vi "Laser manager 1.0BETA.vi"() -> ()   [LabVIEW 2014]
uses:
  <vilib>/userdefined/High Color/IMAQdx.ctl
  Typedef/Consumer loop - States.ctl
  Typedef/UI data.ctl
  <vilib>/vision/driver/NI_Vision_Acquisition_Software.lvlib
panel:
  in  "Move":bool
  in  "Absolute Y":dbl caption="Absolute Y [mm]"
  in  "Absolute X":dbl caption="Absolute X [mm]"
  in  "Delta Y":dbl caption="Delta Y [mm]"
  in  "Delta X":dbl caption="Delta X [mm]"
  in  "Move type":enum32{"Step mode", "\"Go to\" mode"}(radio)=enum."\"Go to\" mode"
  in  "Right":bool
  in  "Left":bool
  in  "Up":bool
  in  "Down":bool
  in  "Exit":bool
  out "Image":T1(plugin-control)
  in  "Tab Control":enum32{"Standard operations", "Refill", "Tools"}(tab)
  in  "Main - Open calib":bool
  in  "Go to calib":bool
  in  "Save calib":bool
  in  "Thyratron Bias [kV]":dbl=20.0
  in  "Test Laser":bool
  in  "Frequency [Hz]":u16=1 min=1 max=50 step=1
  in  "Beam Y":dbl=63.0 caption="Y" min=0.1 step=1.0 format="%#_gmm"
  in  "Beam X":dbl=1.0 caption="X" min=0.1 step=1.0 format="%#_gmm"
  in  "How to choose":bool
  in  "Load Pt2":bool
  out "X2":dbl format="%.2fmm"
  out "Y2":dbl format="%.2fmm"
  in  "Load Pt1":bool
  out "X1":dbl format="%.2fmm"
  out "Y1":dbl format="%.2fmm"
  in  "Abort":bool
  in  "Beam Overlap":dbl caption="Lateral Overlap [mm]" min=0.0 max=62.0 step=1.0
  in  "Shots/point":dbl=1.0 min=1.0 max=200.0 step=1.0
  in  "Xspeed":dbl=1.0 caption="X speed [mm/s]" min=0.01 max=100.0 format="%#_3g"
  in  "Irradiate":bool
  out "Pressure":string caption="Pressure [mbar]"
  in  "Refill":bool
  in  "Purge Inert":bool
  in  "Purge Buffer":bool
  in  "Purge Rare":bool
  in  "Purge Halogen":bool
  in  "Set Gas Pressures [mbar]":T2={"Halogen"=80, "Rare"=60, "Buffer "=3160, "Inert"=0}
  in  "Open GPIB interface":bool
  in  "Enable motors":bool
  in  "Find Origin":bool
  in  "Reset ESP":bool
  in  "Tools - Open Calib":bool
  in  "Open Attenuator":bool
  # "Free mode"
  # "LASER MANAGER 1.0 BETA"
  # "written by frax84"
  # "Energy Calibration"
  # "Laser Parameters"
  # "Beam parameters"
  # "Beam size"
  # "Motor path settings"
  # "Irradiation main controls"
  # "Purge Options"
  # "CAUTION\nEach purge operation \nlasts 5 seconds!"
  # "Reading is performed\nevery 5 seconds"
  # "Peripherals comunication"
  # "Motor Utilities"
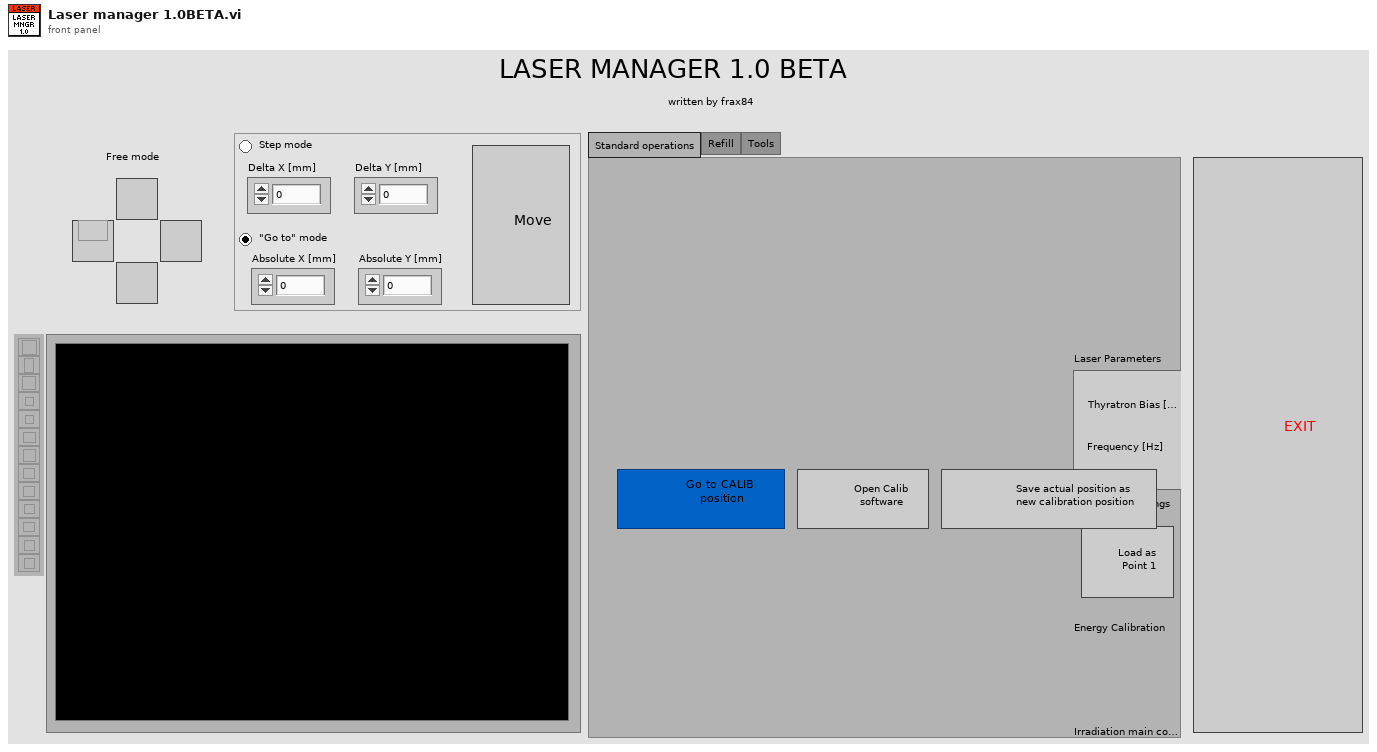
[diagram p1: front panel]
types:
  T1 = typedef "IMAQ Image.ctl" = refnum<image>
  T2 = cluster{"Halogen":u16, "Rare":u16, "Buffer ":u16, "Inert":u16}
  T3 = typedef "UI data.ctl" = cluster{"GPIB Addresses":cluster{"GPIB Motor":i16, "GPIB Laser":string}, "Beam size":cluster{"BeamX":dbl, "BeamY":dbl, "Beam Overlap":dbl}, "Motor speed":cluster{"Xspeed":dbl, " Yspeed":dbl}, "Laser parameters":cluster{"Thyratron Bias":dbl, "Frequency":u16, "Shots/Point":dbl}, "Irradiation points":cluster{"X1":dbl, "Y1":dbl, "X2":dbl, "Y2":dbl}, "Calibration Point":cluster{"Xcalib":dbl, "Ycalib":dbl}}
  T4 = typedef "Consumer loop - States.ctl" = enum16{"Idle", "Read Pressure", "Move up", "Move down", "Move left", "Move right", "Move to", "Move Delta", "Stop Motion", "Go to calib", "Check if move done", "Disable buttons", "Enable buttons", "Irradiation - Stop", "Irradiation - Check points", "Irradiation - Disable buttons", "Irradiation - Init position", "Irradiation - Check if done", "Irradiation - Sweep X", "Irradiation - Check X", "Irradiation - Check Y", "Irradiation - Sweep Y", "Irradiation - Enable buttons"}
  T5 = typedef "Image Type" = u32
  T6 = typedef "IMAQdx.ctl" = refnum<k21>
  T7 = enum8{"Enabled", "Disabled", "Disabled and Grayed Out"}
  T8 = cluster{"Global Rectangle":i32[], "Contours":cluster{"Contour Type":u32, "ROI Type":u32, "Points":i32[]}[]}
  T9 = cluster{"Global Rectangle[0]":i32, "Global Rectangle[1]":i32, "Global Rectangle[2]":i32, "Global Rectangle[3]":i32}
  T10 = cluster{"Consumer loop - States":T4, "Variant":variant}
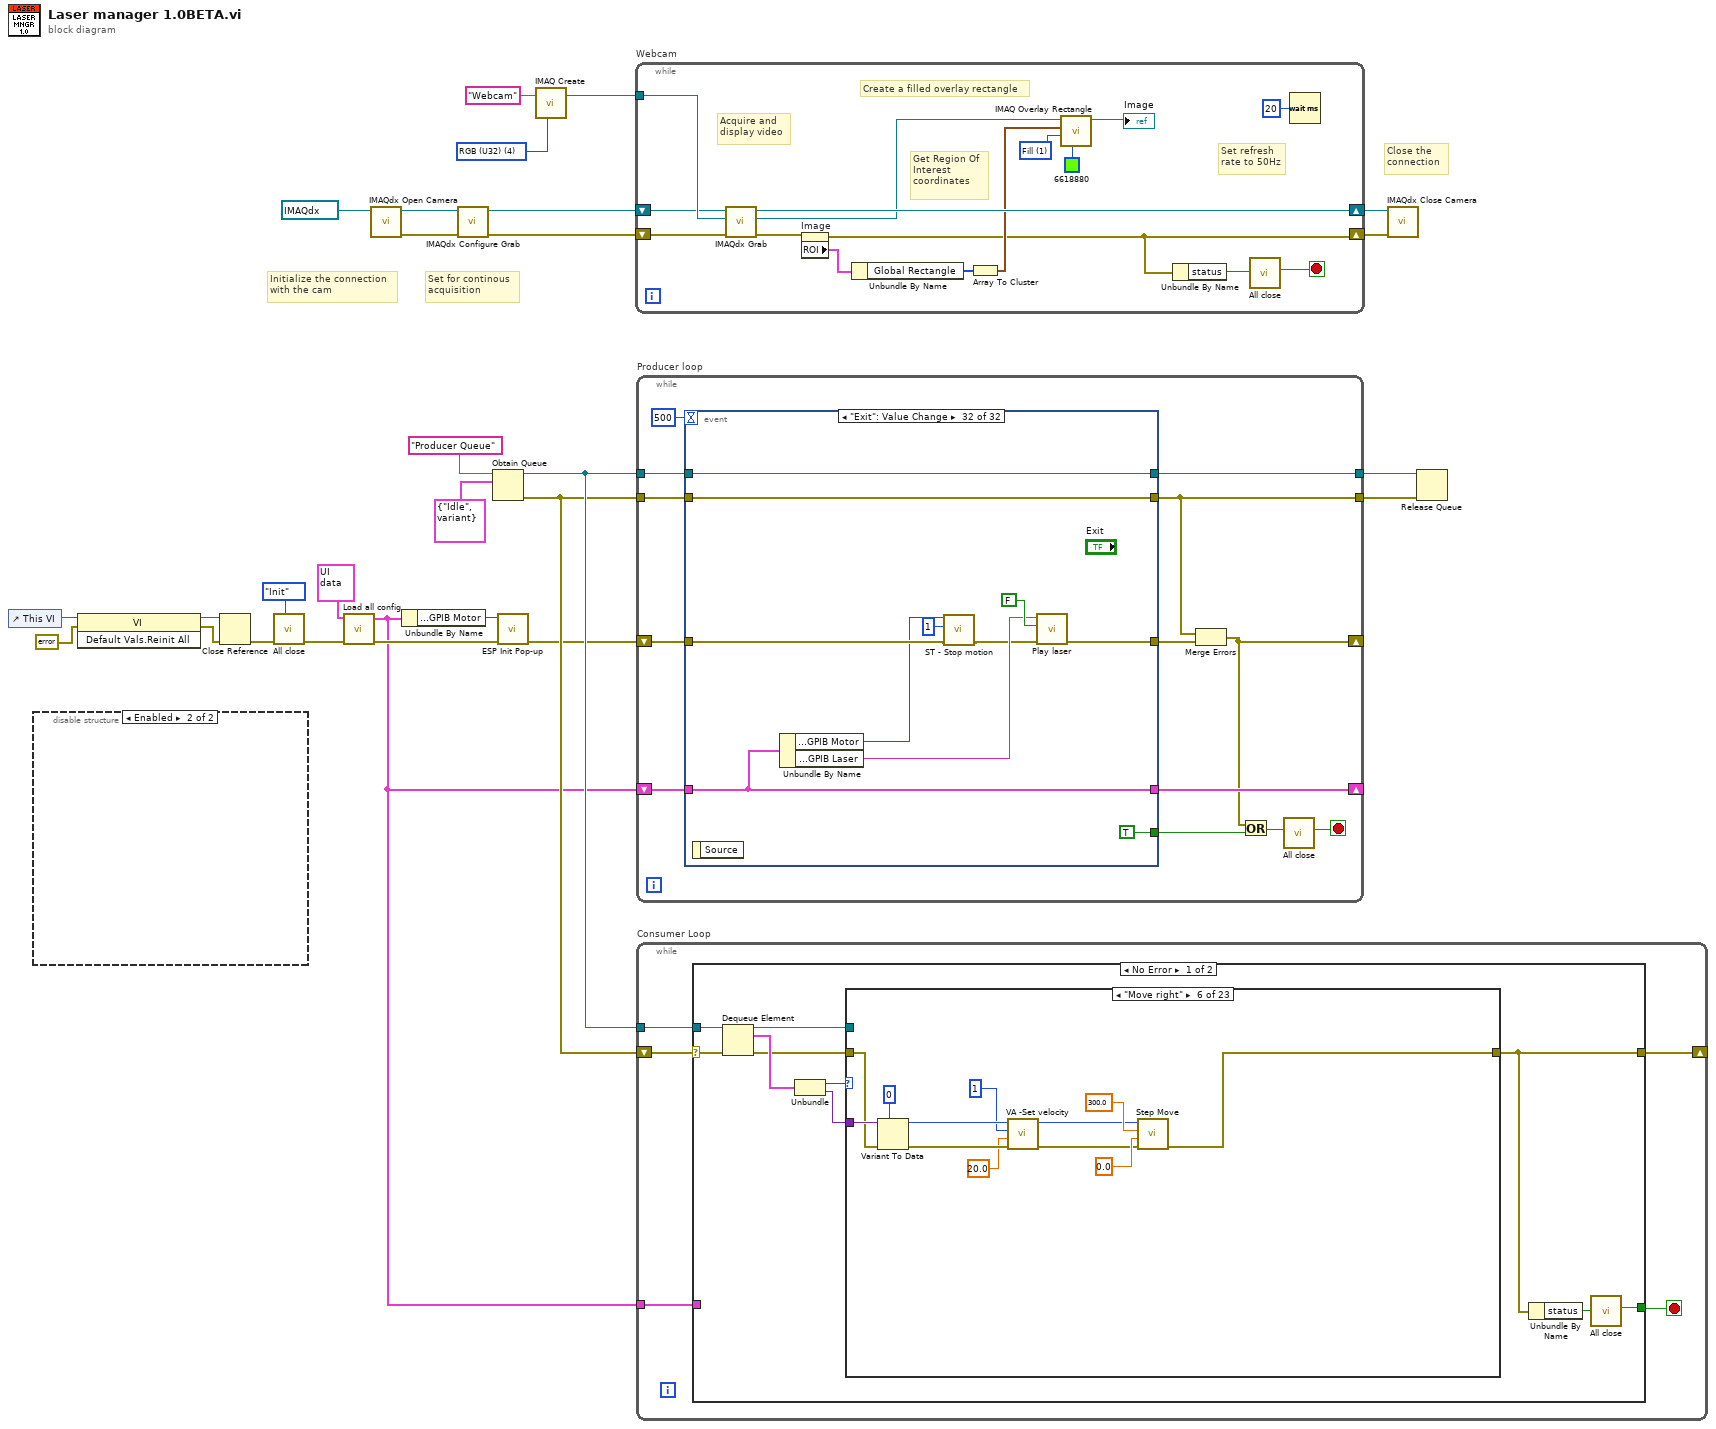
[diagram p0: block diagram]
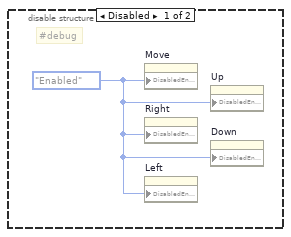
[diagram p2: hidden frame]
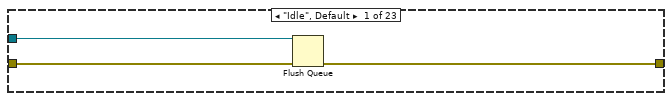
[diagram p3: hidden frame]
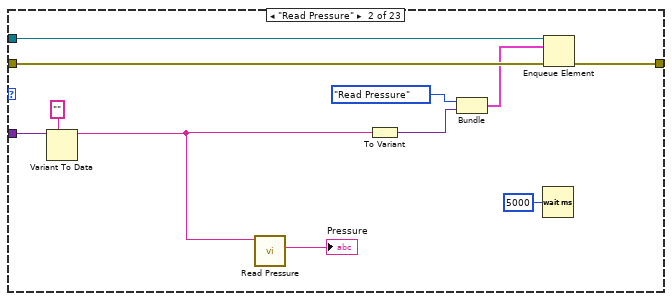
[diagram p4: hidden frame]
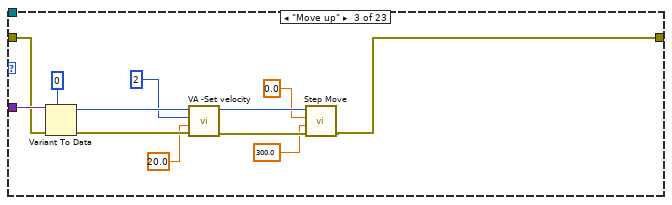
[diagram p5: hidden frame]
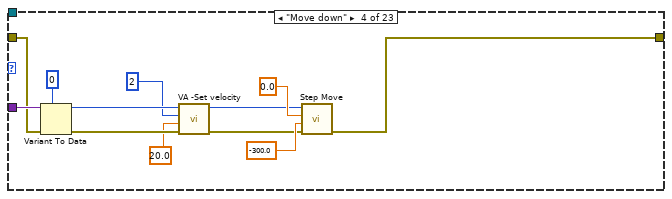
[diagram p6: hidden frame]
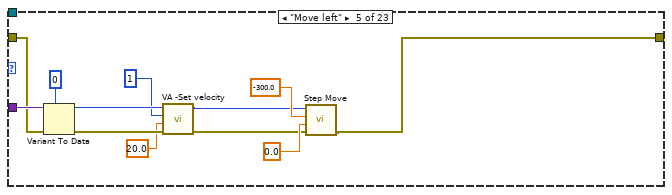
[diagram p7: hidden frame]
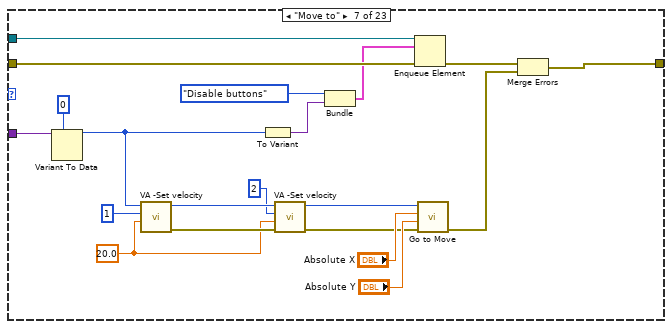
[diagram p8: hidden frame]
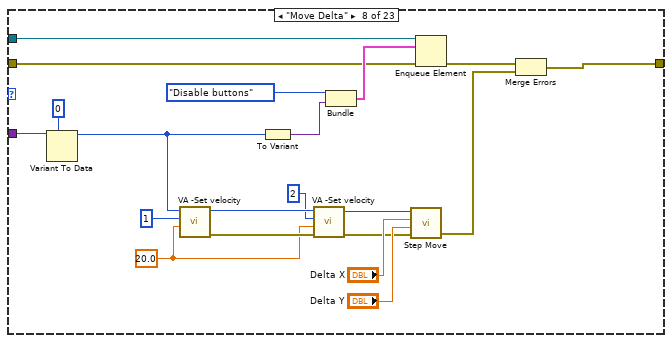
[diagram p9: hidden frame]
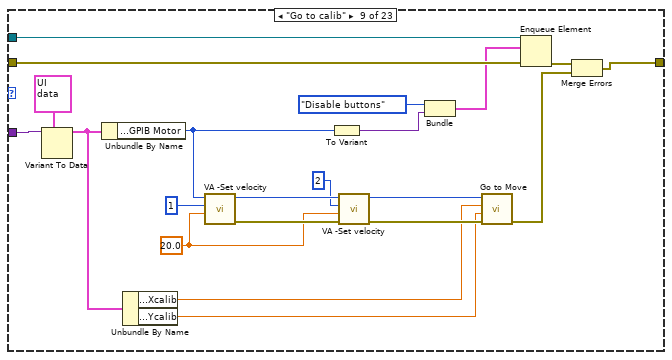
[diagram p10: hidden frame]
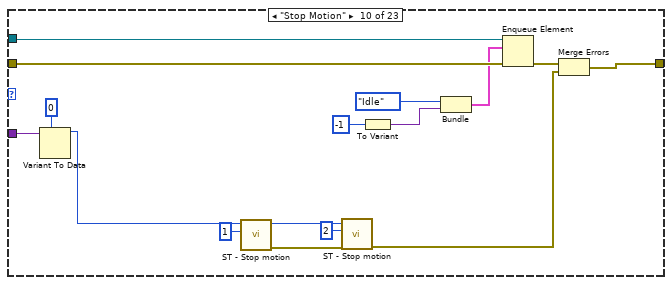
[diagram p11: hidden frame]
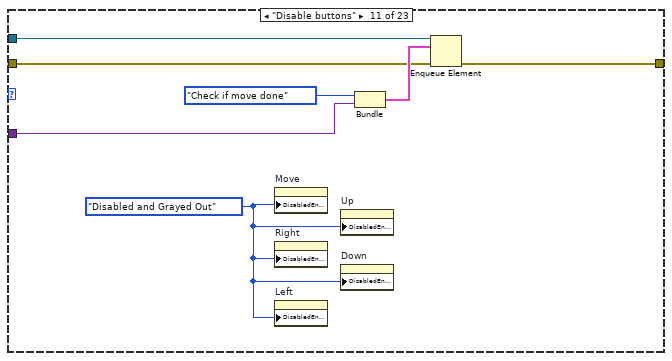
[diagram p12: hidden frame]
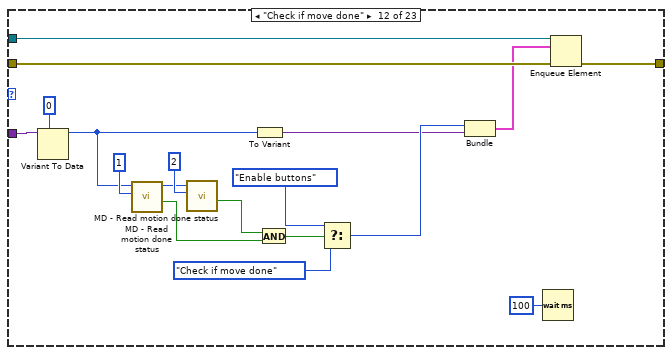
[diagram p13: hidden frame]
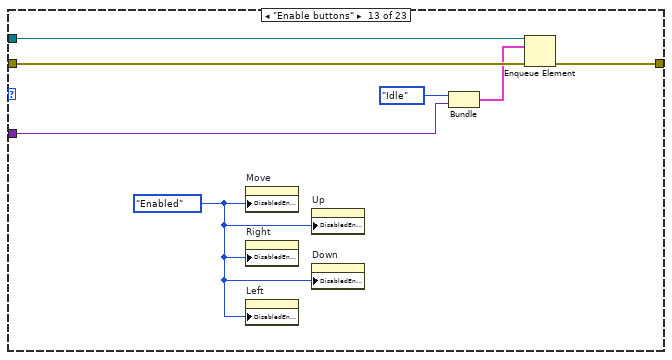
[diagram p14: hidden frame]
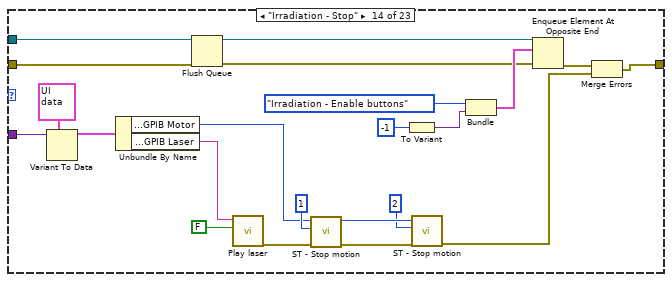
[diagram p15: hidden frame]
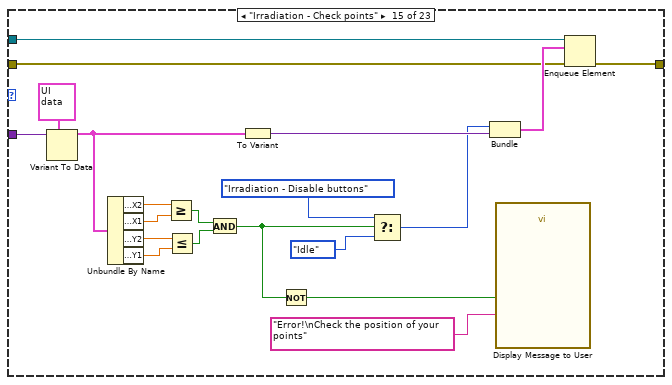
[diagram p16: hidden frame]
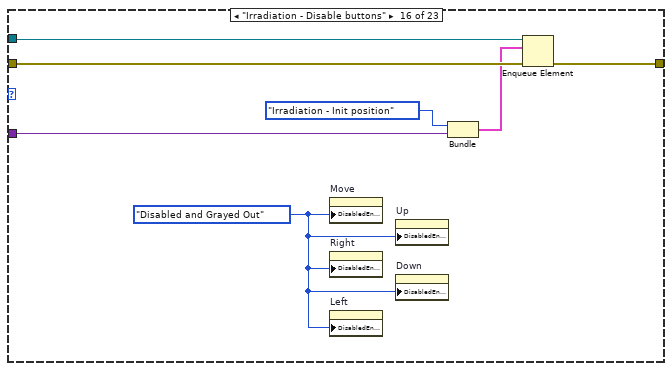
[diagram p17: hidden frame]
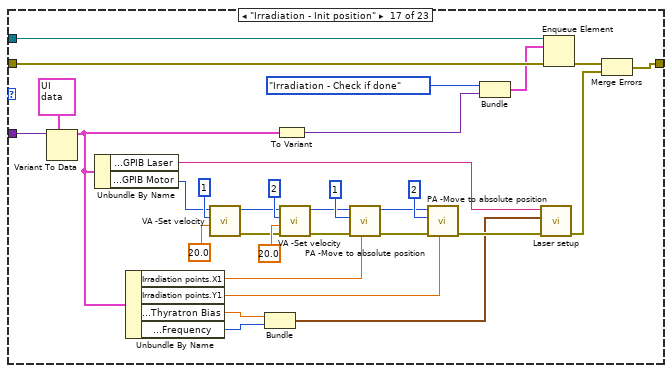
[diagram p18: hidden frame]
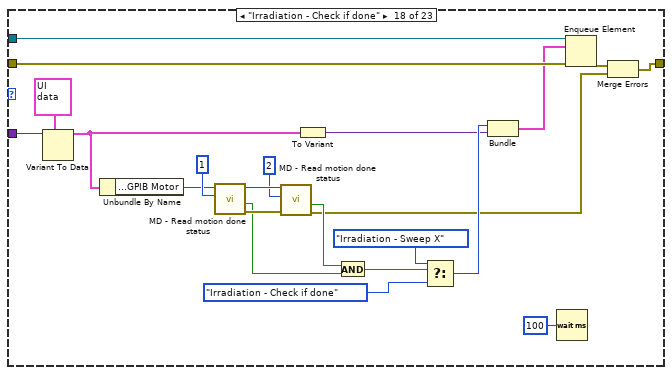
[diagram p19: hidden frame]
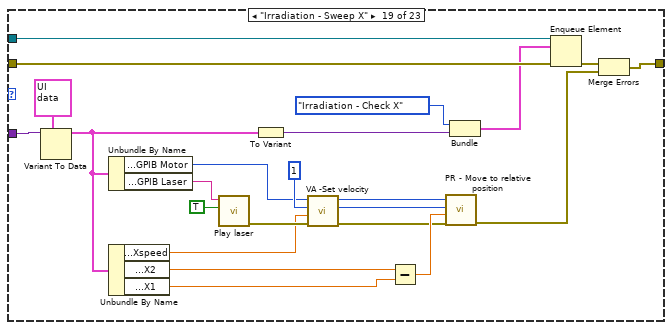
[diagram p20: hidden frame]
diagram:
  w22 = T5 4 items=["Grayscale (U8)", "Grayscale (I16)", "Grayscale (SGL)", "Complex (CSG)", "RGB (U32)", "HSL (U32)", "RGB (U64)", "Grayscale (U16)"] ("Image Type")
  # "Close the \nconnection"
  # "Set for continous\nacquisition"
  # "Initialize the connection\nwith the cam"
  n1 = control-ref of="This VI"() -> (w5:refnum<vi>)
  n2 = disable-structure shown="Enabled" {
    frame Disabled {
      w29 = T7."Enabled" ("Disabled")
      # "#debug"
      n3 = property on="Move" class="Bool"("DisabledEnum"=w29) -> ()  [unwired: 2 in, 2 out]
      n4 = property on="Right" class="Bool (strict)"("DisabledEnum"=w29) -> ()  [unwired: 2 in, 2 out]
      n5 = property on="Left" class="Bool (strict)"("DisabledEnum"=w29) -> ()  [unwired: 2 in, 2 out]
      n6 = property on="Up" class="Bool (strict)"("DisabledEnum"=w29) -> ()  [unwired: 2 in, 2 out]
      n7 = property on="Down" class="Bool (strict)"("DisabledEnum"=w29) -> ()  [unwired: 2 in, 2 out]
    }
    frame Enabled {
    }
  }
  n8 = invoke class="VI" method="Default Vals.Reinit All"(reference=w5, error in=errorcluster {"status"=FALSE, "code"=0, "source"=""} ("Error In")) -> (reference out=w3:refnum<vi>, error out=w4:errorcluster)  [unwired: 1 in, 1 out]
  n9 = Close Reference(reference=w3, error in (no error)=w4) -> (error out=w2:errorcluster)
  n10 = call "All close.vi"("Operation (Check)"=enum16{"Init", "Check"}."Init" ("Operation"), "Error In"=w2) -> ("Error Out"=w8:errorcluster)  [unwired: 8 in, 1 out]
  n11 = call "Load all config.vi"("Error In"=w8, "UI data in"=T3 {"GPIB Addresses"={"GPIB Motor"=2, "GPIB Laser"="3"}, "Beam size"={"BeamX"=1.0, "BeamY"=63.0, "Beam Overlap"=0.0}, "Motor speed"={"Xspeed"=1.0, " Yspeed"=1.0}, "Laser parameters"={"Thyratron Bias"=20.0, "Frequency"=1, "Shots/Point"=1.0}, "Irradiation points"={"X1"=0.0, "Y1"=0.0, "X2"=0.0, "Y2"=0.0}, "Calibration Point"={"Xcalib"=0.0, "Ycalib"=0.0}} ("User Interface data")) -> ("Error Out"=w10:errorcluster, "UI data out"=w9:T3)  [unwired: 8 in]
  n12 = call <vilib>:"IMAQdx Open Camera.vi"("Session In"=T6 "cam1") -> ("error out"=w27:errorcluster, "Session Out"=w28:T6)  [unwired: 9 in]
  n13 = Unbundle By Name(w9) -> ("GPIB Addresses.GPIB Motor"=w13:i16)
  n14 = call <vilib>:"IMAQdx Configure Grab.vi"("error in"=w27, "Session In"=w28) -> ("error out"=w20:errorcluster, "Session Out"=w19:T6)  [unwired: 8 in]
  n15 = Obtain Queue(name (unnamed)="Producer Queue", element data type=cluster{"Consumer loop - States":T4, variant} {"Consumer loop - States"=enum."Idle", variant}) -> (queue out=w17:refnum<queue>, error out=w16:errorcluster)  [unwired: 3 in, 1 out]
  n16 = call "ESP Init Pop-up.vi"("Error In"=w10, "Address / Port in"=w13) -> ("Error Out"=w14:errorcluster)  [unwired: 9 in]
  n17 = call "IMAQ Create"("Image Name"="Webcam", "Image Type"=w22) -> ("New Image"=w23:T1)  [unwired: 3 in, 1 out]
  n18 = while "Webcam" {
    shift-right: [w45] -> w25
    shift-left: w19 -> [w43]
    shift-right: [w31] -> w24
    shift-left: w20 -> [w42]
    tunnel: w23 -> [w44]
    stop <- w32 stop-if-true
    w35 = u32 1 items=["Frame", "Fill", "Highlight"] ("Drawing Mode (Frame)")
    # "Set refresh \nrate to 50Hz"
    # "Get Region Of \nInterest\ncoordinates"
    # "Create a filled overlay rectangle"
    # "Acquire and \ndisplay video"
    n19 = call <vilib>:"IMAQdx Grab.vi"("error in"=w42, "Image In"=w44, "Session In"=w43) -> ("error out"=w41:errorcluster, "Image Out"=w36:T1, "Session Out"=w45:T6)  [unwired: 5 in, 1 out]
    n20 = property on="Image" class="ImageControl"(error in=w41) -> (error out=w31:errorcluster, "ROI"=w40:T8)  [unwired: 1 in, 1 out]
    n21 = Unbundle By Name(w40) -> ("Global Rectangle"=w39:i32[])
    n22 = Array To Cluster(array=w39) -> (cluster=w38:T9)
    n23 = call "IMAQ Overlay Rectangle"("Color"=u32 6618880, "Drawing Mode (Frame)"=w35, "Rectangle"=w38, "Image"=w36) -> ("Image Out"=→"Image":T1)  [unwired: 6 in, 1 out]
    n24 = Unbundle By Name(w31) -> ("status"=w30:bool)
    n25 = call "All close.vi"("Close? (F)"=w30) -> ("Close"=w32:bool)  [unwired: 9 in, 1 out]
    n26 = Wait (ms)(milliseconds to wait=u32 20) -> ()  [unwired: 1 out]
  }
  n27 = while "Producer loop" {
    shift-right: [w49] -> _
    shift-left: w14 -> [w58]
    shift-right: [w56] -> _
    shift-left: w9 -> [w57]
    tunnel: w17 -> [w54]
    tunnel: w16 -> [w53]
    tunnel: [w48] -> w12
    tunnel: [w51] -> w11
    stop <- w46 stop-if-true
    n28 = event shown="[31] \"Exit\": Value Change" {
      selector: _ -> [_ _ _ _ _ _ _ _ _ _ _ _ _ _ _ _ _ _ _ _ _ _ _ _ _ _ _ _ _ _ _ _]
      dyn-events: _ -> [_ _ _ _ _ _ _ _ _ _ _ _ _ _ _ _ _ _ _ _ _ _ _ _ _ _ _ _ _ _ _ _]
      timeout: 500 -> [_ _ _ _ _ _ _ _ _ _ _ _ _ _ _ _ _ _ _ _ _ _ _ _ _ _ _ _ _ _ _ _]
      tunnel: w58 -> [w62 w77 w78 w91 w104 w117 w134 w153 w162 w175 w188 w198 w204 w225 w235 w245 w250 w260 w265 w274 w280 w287 w296 w305 w313 w321 w328 w336 w341 w365 w374 w380]
      tunnel: [w62 w77 w78 w91 w104 w117 w134 w141 w161 w174 w187 w197 w204 w225 w235 w245 w250 w260 w265 w273 w279 w286 w295 w304 w312 w320 w326 w337 w341 w365 w373 w384] -> w50
      tunnel: w57 -> [w61 w68 w83 w97 w108 w123 w131 w147 w159 w172 w182 w192 w200 w224 w231 w241 w253 w259 w268 w271 w277 w284 w294 w303 w311 w318 w327 w335 w345 w362 w372 w385]
      tunnel: [w61 w68 w83 w97 w108 w123 w131 w142 w156 w171 w182 w192 w200 w224 w229 w239 w251 w258 w266 w271 w277 w284 w294 w303 w311 w318 w327 w335 w345 w362 w372 w385] -> w56
      tunnel: [_ _ _ _ _ _ _ _ _ _ _ _ _ _ _ _ _ _ _ _ _ _ _ _ _ _ _ _ _ _ _ TRUE] -> w52
      tunnel: w54 -> [w60 w76 w87 w96 w110 w122 w138 w139 w155 w168 w181 w191 w211 w222 w228 w238 w249 w262 w264 w270 w276 w283 w289 w301 w309 w317 w325 w333 w353 w364 w369 w381]
      tunnel: w53 -> [w59 w75 w86 w95 w109 w121 w135 w140 w154 w167 w180 w190 w212 w223 w227 w237 w248 w261 w263 w269 w275 w282 w288 w300 w308 w316 w324 w332 w352 w363 w367 w382]
      tunnel: [w59 w63 w79 w92 w105 w118 w136 w140 w154 w167 w180 w190 w212 w223 w227 w237 w248 w261 w263 w269 w275 w282 w288 w300 w308 w316 w324 w332 w339 w358 w366 w382] -> w48
      tunnel: [w60 w64 w80 w93 w106 w119 w137 w139 w155 w168 w181 w191 w211 w222 w228 w238 w249 w262 w264 w270 w276 w283 w289 w301 w309 w317 w325 w333 w340 w359 w368 w381] -> w51
      event Timeout {
        # "Needed if error occurs"
        n29 = event-data() -> ()  [unwired: 1 in, 1 out]
      }
      event "Move": Value Change {
        n30 = event-data() -> ()  [unwired: 1 in, 1 out]
        n31 = Unbundle By Name(w68) -> ("GPIB Addresses.GPIB Motor"=w67:i16)
        n32 = Equal?(x="Move type", y=enum32{"Step mode", "\"Go to\" mode"}."\"Go to\" mode") -> (x = y?=w72:bool)
        n33 = To Variant(anything=w67) -> (Variant=w66:variant)
        n34 = Select(t=Consumer_loop_-_States."Move to" ("Consumer loop - States"), s=w72, f=Consumer_loop_-_States."Move Delta") -> (s? t:f=w71:T4)
        n35 = Bundle("f"=w71, "Variant"=w66) -> (w65:cluster{"f":T4, "Variant":variant})  [unwired: 1 in]
        n36 = Enqueue Element(queue=w76, element=w65, error in (no error)=w75) -> (queue out=w64:refnum<queue>, error out=w63:errorcluster)  [unwired: 1 in, 1 out]
      }
      event "Up": Value Change {
        n37 = event-data() -> ("NewVal"=w90:bool)  [unwired: 1 in]
        n38 = Unbundle By Name(w83) -> ("GPIB Addresses.GPIB Motor"=w81:i16)
        n39 = To Variant(anything=w81) -> (Variant=w82:variant)
        n40 = Select(t=Consumer_loop_-_States."Move up", s=w90, f=Consumer_loop_-_States."Stop Motion" ("Consumer loop - States")) -> (s? t:f=w85:T4)
        n41 = Bundle("Consumer loop - States"=w85, "Variant"=w82) -> (w84:T10)  [unwired: 1 in]
        n42 = Enqueue Element(queue=w87, element=w84, error in (no error)=w86) -> (queue out=w80:refnum<queue>, error out=w79:errorcluster)  [unwired: 1 in, 1 out]
      }
      event "Down": Value Change {
        n43 = event-data() -> ("NewVal"=w94:bool)  [unwired: 1 in]
        n44 = Unbundle By Name(w97) -> ("GPIB Addresses.GPIB Motor"=w98:i16)
        n45 = To Variant(anything=w98) -> (Variant=w99:variant)
        n46 = Select(t=Consumer_loop_-_States."Move down", s=w94, f=Consumer_loop_-_States."Stop Motion" ("Consumer loop - States")) -> (s? t:f=w101:T4)
        n47 = Bundle("Consumer loop - States"=w101, "Variant"=w99) -> (w100:T10)  [unwired: 1 in]
        n48 = Enqueue Element(queue=w96, element=w100, error in (no error)=w95) -> (queue out=w93:refnum<queue>, error out=w92:errorcluster)  [unwired: 1 in, 1 out]
      }
      event "Left": Value Change {
        n49 = event-data() -> ("NewVal"=w107:bool)  [unwired: 1 in]
        n50 = Unbundle By Name(w108) -> ("GPIB Addresses.GPIB Motor"=w116:i16)
        n51 = To Variant(anything=w116) -> (Variant=w115:variant)
        n52 = Select(t=Consumer_loop_-_States."Move left", s=w107, f=Consumer_loop_-_States."Stop Motion" ("Consumer loop - States")) -> (s? t:f=w113:T4)
        n53 = Bundle("Consumer loop - States"=w113, "Variant"=w115) -> (w114:T10)  [unwired: 1 in]
        n54 = Enqueue Element(queue=w110, element=w114, error in (no error)=w109) -> (queue out=w106:refnum<queue>, error out=w105:errorcluster)  [unwired: 1 in, 1 out]
      }
      event "Right": Value Change {
        n55 = event-data() -> ("NewVal"=w120:bool)  [unwired: 1 in]
        n56 = Unbundle By Name(w123) -> ("GPIB Addresses.GPIB Motor"=w129:i16)
        n57 = To Variant(anything=w129) -> (Variant=w128:variant)
        n58 = Select(t=Consumer_loop_-_States."Move right", s=w120, f=Consumer_loop_-_States."Stop Motion" ("Consumer loop - States")) -> (s? t:f=w126:T4)
        n59 = Bundle("Consumer loop - States"=w126, "Variant"=w128) -> (w127:T10)  [unwired: 1 in]
        n60 = Enqueue Element(queue=w122, element=w127, error in (no error)=w121) -> (queue out=w119:refnum<queue>, error out=w118:errorcluster)  [unwired: 1 in, 1 out]
      }
      event "Go to calib": Value Change {
        n61 = event-data() -> ()  [unwired: 1 in, 1 out]
        n62 = To Variant(anything=w131) -> (Variant=w130:variant)
        n63 = Bundle("Consumer loop - States"=Consumer_loop_-_States."Go to calib", "Variant"=w130) -> (w133:T10)  [unwired: 1 in]
        n64 = Enqueue Element(queue=w138, element=w133, error in (no error)=w135) -> (queue out=w137:refnum<queue>, error out=w136:errorcluster)  [unwired: 1 in, 1 out]
      }
      event "Save calib": Value Change {
        n65 = event-data() -> ()  [unwired: 1 in, 1 out]
        n66 = Unbundle By Name(w147) -> ("GPIB Addresses.GPIB Motor"=w152:i16)
        n67 = call "TP - Read actual position.vi"("error in"=w153, "Axis"=i8 1, "Address / Port"=w152) -> ("error out"=w150:errorcluster, "Query the current actual\nposition - read"=w146:dbl, "Address / Port dup"=w149:i16)  [unwired: 5 in, 1 out]
        n68 = call "TP - Read actual position.vi"("error in"=w150, "Axis"=i8 2, "Address / Port"=w149) -> ("error out"=w144:errorcluster, "Query the current actual\nposition - read"=w145:dbl)  [unwired: 5 in, 2 out]
        n69 = Bundle By Name(cluster=w147, "Calibration Point.Ycalib"=w145, "Calibration Point.Xcalib"=w146) -> (w143:T3)
        n70 = call "Save calib config.vi"("Error In"=w144, "UI data in"=w143) -> ("Error Out"=w141:errorcluster, "UI data out"=w142:T3)  [unwired: 8 in]
      }
      event "Load Pt1": Value Change {
        n71 = event-data() -> ()  [unwired: 1 in, 1 out]
        n72 = Unbundle By Name(w159) -> ("GPIB Addresses.GPIB Motor"=w160:i16)
        n73 = call "TP - Read actual position.vi"("error in"=w162, "Axis"=i8 1, "Address / Port"=w160) -> ("error out"=w165:errorcluster, "Query the current actual\nposition - read"=w158:dbl, "Address / Port dup"=w166:i16)  [unwired: 5 in, 1 out]
        "X1" <- w158
        n74 = call "TP - Read actual position.vi"("error in"=w165, "Axis"=i8 2, "Address / Port"=w166) -> ("error out"=w161:errorcluster, "Query the current actual\nposition - read"=w157:dbl)  [unwired: 5 in, 2 out]
        "Y1" <- w157
        n75 = Bundle By Name(cluster=w159, "Irradiation points.Y1"=w157, "Irradiation points.X1"=w158) -> (w156:T3)
      }
      event "Load Pt2": Value Change {
        n76 = event-data() -> ()  [unwired: 1 in, 1 out]
        n77 = Unbundle By Name(w172) -> ("GPIB Addresses.GPIB Motor"=w173:i16)
        n78 = call "TP - Read actual position.vi"("error in"=w175, "Axis"=i8 1, "Address / Port"=w173) -> ("error out"=w178:errorcluster, "Query the current actual\nposition - read"=w170:dbl, "Address / Port dup"=w179:i16)  [unwired: 5 in, 1 out]
        "X2" <- w170
        n79 = call "TP - Read actual position.vi"("error in"=w178, "Axis"=i8 2, "Address / Port"=w179) -> ("error out"=w174:errorcluster, "Query the current actual\nposition - read"=w169:dbl)  [unwired: 5 in, 2 out]
        "Y2" <- w169
        n80 = Bundle By Name(cluster=w172, "Irradiation points.Y2"=w169, "Irradiation points.X2"=w170) -> (w171:T3)
      }
      event "Tools - Open Calib", "Main - Open calib": Value Change {
        n81 = event-data() -> ()  [unwired: 1 in, 1 out]
        n82 = call <vilib>:"Application Directory.vi"() -> ("Application Directory"=w186:path)
        n83 = Build Path(base path=w186, name or relative path="External software\\Thorlabs\\Optical Power Meter Utility.exe" ("command line")) -> (appended path=w185:path)
        n84 = Path To String(path=w185) -> (string=w183:string)
        n85 = call <vilib>:"System Exec.vi"("wait until completion? (T)"=FALSE, "error in (no error)"=w188, "command line"=w183) -> ("error out"=w187:errorcluster)  [unwired: 5 in, 3 out]
      }
      event "Open Attenuator": Value Change {
        n86 = event-data() -> ()  [unwired: 1 in, 1 out]
        n87 = call <vilib>:"Application Directory.vi"() -> ("Application Directory"=w196:path)
        n88 = Build Path(base path=w196, name or relative path="External software\\Coherent\\CohrAttenuatorApp.exe" ("command line")) -> (appended path=w195:path)
        n89 = Path To String(path=w195) -> (string=w193:string)
        n90 = call <vilib>:"System Exec.vi"("wait until completion? (T)"=FALSE, "error in (no error)"=w198, "command line"=w193) -> ("error out"=w197:errorcluster)  [unwired: 5 in, 3 out]
      }
      event "Open GPIB interface": Value Change {
        n91 = event-data() -> ()  [unwired: 1 in, 1 out]
        n92 = call <vilib>:"Application Directory.vi"() -> ("Application Directory"=w203:path)
        n93 = Build Path(base path=w203, name or relative path="Utilities\\GPIB \nSimple Interface.vi") -> (appended path=w201:path)
        n94 = Open VI Reference(vi path=w201) -> (vi reference=w209:refnum<vi>, error out=w206:errorcluster)  [unwired: 5 in]
        n95 = property class="VI"(reference=w209, error in=w206, "Front Panel Window:Open"=TRUE) -> (reference out=w208:refnum<vi>, error out=w205:errorcluster)
        n96 = invoke class="VI" method="Run VI"(reference=w208, error in=w205, "Wait until done"=FALSE) -> ()  [unwired: 2 in, 5 out]
      }
      event "How to choose": Value Change {
        n97 = event-data() -> ()  [unwired: 1 in, 1 out]
        n98 = call <vilib>:"Application Directory.vi"() -> ("Application Directory"=w215:path)
        n99 = Build Path(base path=w215, name or relative path="SubVIs\\How to.vi") -> (appended path=w213:path)
        n100 = Open VI Reference(vi path=w213) -> (vi reference=w220:refnum<vi>, error out=w217:errorcluster)  [unwired: 5 in]
        n101 = property class="VI"(reference=w220, error in=w217, "Front Panel Window:Open"=TRUE) -> (reference out=w219:refnum<vi>, error out=w216:errorcluster)
        n102 = invoke class="VI" method="Run VI"(reference=w219, error in=w216, "Wait until done"=FALSE) -> ()  [unwired: 2 in, 5 out]
      }
      event "Shots/point": Value Change {
        n103 = event-data() -> ()  [unwired: 1 in, 1 out]
        n104 = Unbundle By Name(w231) -> ("Beam size.BeamX"=w234:dbl, "Laser parameters.Frequency"=w233:u16)
        n105 = Multiply(x=w234, y=w233) -> (x*y=w232:dbl)
        n106 = Divide(x=w232, y="Shots/point") -> (x/y=w226:dbl)
        n107 = Bundle By Name(cluster=w231, "Motor speed.Xspeed"=w226, "Laser parameters.Shots/Point"="Shots/point") -> (w229:T3)
        n108 = local write "Xspeed"(w226) -> ()
      }
      event "Xspeed": Value Change {
        n109 = event-data() -> ()  [unwired: 1 in, 1 out]
        n110 = Unbundle By Name(w241) -> ("Beam size.BeamX"=w244:dbl, "Laser parameters.Frequency"=w243:u16)
        n111 = Multiply(x=w244, y=w243) -> (x*y=w242:dbl)
        n112 = Divide(x=w242, y="Xspeed") -> (x/y=w236:dbl)
        n113 = local write "Shots/point"(w236) -> ()
        n114 = Bundle By Name(cluster=w241, "Laser parameters.Shots/Point"=w236, "Motor speed.Xspeed"="Xspeed") -> (w239:T3)
      }
      event "Frequency [Hz]", "Beam X": Value Change {
        n115 = event-data() -> ()  [unwired: 1 in, 1 out]
        n116 = Unbundle By Name(w253) -> ("Laser parameters.Shots/Point"=w254:dbl)
        n117 = Multiply(x="Frequency [Hz]", y="Beam X") -> (x*y=w255:dbl)
        n118 = Divide(x=w255, y=w254) -> (x/y=w247:dbl)
        n119 = local write "Xspeed"(w247) -> ()
        n120 = Bundle By Name(cluster=w253, "Laser parameters.Frequency"="Frequency [Hz]", "Beam size.BeamX"="Beam X", "Motor speed.Xspeed"=w247) -> (w251:T3)
      }
      event "Beam Overlap", "Beam Y": Value Change {
        n121 = event-data() -> ()  [unwired: 1 in, 1 out]
        n122 = Bundle By Name(cluster=w259, "Beam size.BeamY"="Beam Y", "Beam size.Beam Overlap"="Beam Overlap") -> (w258:T3)
      }
      event "Thyratron Bias [kV]": Value Change {
        n123 = event-data() -> ()  [unwired: 1 in, 1 out]
        n124 = Bundle By Name(cluster=w268, "Laser parameters.Thyratron Bias"="Thyratron Bias [kV]") -> (w266:T3)
      }
      event "Find Origin": Value Change {
        n125 = event-data() -> ()  [unwired: 1 in, 1 out]
        n126 = Unbundle By Name(w271) -> ("GPIB Addresses.GPIB Motor"=w272:i16)
        n127 = call "Find Origin.vi"("Error In"=w274, "Address / Port"=w272) -> ("Error Out"=w273:errorcluster)  [unwired: 8 in, 1 out]
      }
      event "Enable motors": Value Change {
        n128 = event-data() -> ()  [unwired: 1 in, 1 out]
        n129 = Unbundle By Name(w277) -> ("GPIB Addresses.GPIB Motor"=w278:i16)
        n130 = call "Enable Motor.vi"("Error In"=w280, "On/Off"=enum16{"On", "Off"}."On", "Address / Port"=w278) -> ("Error Out"=w279:errorcluster)  [unwired: 7 in, 1 out]
      }
      event "Reset ESP": Value Change {
        n131 = event-data() -> ()  [unwired: 1 in, 1 out]
        n132 = Unbundle By Name(w284) -> ("GPIB Addresses.GPIB Motor"=w285:i16)
        n133 = call "RS - Reset the controller.vi"("error in"=w287, "Address / Port"=w285) -> ("error out"=w286:errorcluster)  [unwired: 6 in, 1 out]
      }
      event "Test Laser": Value Change {
        n134 = event-data() -> ("NewVal"=w297:bool)  [unwired: 1 in]
        n135 = Unbundle By Name(w294) -> ("GPIB Addresses.GPIB Laser"=w293:string, "Laser parameters.Thyratron Bias"=w292:dbl, "Laser parameters.Frequency"=w291:u16)
        n136 = Bundle("Thyratron Bias"=w292, "Frequency"=w291) -> (w290:cluster{"Thyratron Bias":dbl, "Frequency":u16})  [unwired: 1 in]
        n137 = call "Laser setup.vi"("Error In"=w296, "Laser Parameters"=w290, "GPIB Address"=w293) -> ("Error Out"=w298:errorcluster, "GPIB Address out"=w299:string)  [unwired: 7 in]
        n138 = call "Play laser.vi"("Error In"=w298, "Laser On"=w297, "GPIB Address"=w299) -> ("Error Out"=w295:errorcluster)  [unwired: 7 in, 1 out]
      }
      event "Purge Halogen": Value Change {
        n139 = event-data() -> ()  [unwired: 1 in, 1 out]
        n140 = Unbundle By Name(w303) -> ("GPIB Addresses.GPIB Laser"=w302:string)
        n141 = call "Purge Line.vi"("Error In"=w305, "Gas"=enum16{"Halogen", "Rare", "Buffer", "Inert"}."Halogen", "GPIB Address"=w302) -> ("Error Out"=w304:errorcluster)  [unwired: 7 in, 1 out]
        n142 = Wait (ms)(milliseconds to wait=u32 6000) -> ()  [unwired: 1 out]
      }
      event "Purge Rare": Value Change {
        n143 = event-data() -> ()  [unwired: 1 in, 1 out]
        n144 = Unbundle By Name(w311) -> ("GPIB Addresses.GPIB Laser"=w310:string)
        n145 = call "Purge Line.vi"("Error In"=w313, "Gas"=enum16{"Halogen", "Rare", "Buffer", "Inert"}."Rare", "GPIB Address"=w310) -> ("Error Out"=w312:errorcluster)  [unwired: 7 in, 1 out]
        n146 = Wait (ms)(milliseconds to wait=u32 6000) -> ()  [unwired: 1 out]
      }
      event "Purge Buffer": Value Change {
        n147 = event-data() -> ()  [unwired: 1 in, 1 out]
        n148 = Unbundle By Name(w318) -> ("GPIB Addresses.GPIB Laser"=w319:string)
        n149 = call "Purge Line.vi"("Error In"=w321, "Gas"=enum16{"Halogen", "Rare", "Buffer", "Inert"}."Buffer", "GPIB Address"=w319) -> ("Error Out"=w320:errorcluster)  [unwired: 7 in, 1 out]
        n150 = Wait (ms)(milliseconds to wait=u32 6000) -> ()  [unwired: 1 out]
      }
      event "Purge Inert": Value Change {
        n151 = event-data() -> ()  [unwired: 1 in, 1 out]
        n152 = Unbundle By Name(w327) -> ("GPIB Addresses.GPIB Laser"=w329:string)
        n153 = call "Purge Line.vi"("Error In"=w328, "Gas"=enum16{"Halogen", "Rare", "Buffer", "Inert"}."Inert", "GPIB Address"=w329) -> ("Error Out"=w326:errorcluster)  [unwired: 7 in, 1 out]
        n154 = Wait (ms)(milliseconds to wait=u32 6000) -> ()  [unwired: 1 out]
      }
      event "Refill": Value Change {
        n155 = event-data() -> ()  [unwired: 1 in, 1 out]
        n156 = Unbundle By Name(w335) -> ("GPIB Addresses.GPIB Laser"=w334:string)
        n157 = call "New Fill.vi"("Error In"=w336, "Gas settings"="Set Gas Pressures [mbar]", "GPIB Address"=w334) -> ("Error Out"=w337:errorcluster)  [unwired: 7 in, 1 out]
      }
      event "Tab Control": Value Change {
        # "If the Refill tab is chosen pressure is read every 5 seconds"
        n158 = event-data() -> ()  [unwired: 1 in, 1 out]
        n159 = Unbundle By Name(w345) -> ("GPIB Addresses.GPIB Laser"=w344:string)
        n160 = Equal?(x="Tab Control", y=enum32{"Standard operations", "Refill", "Tools"}."Refill") -> (x = y?=w349:bool)
        n161 = To Variant(anything=w344) -> (Variant=w343:variant)
        n162 = Select(t=Consumer_loop_-_States."Read Pressure" ("Consumer loop - States"), s=w349, f=Consumer_loop_-_States."Idle") -> (s? t:f=w346:T4)
        n163 = Bundle("f"=w346, "Variant"=w343) -> (w342:cluster{"f":T4, "Variant":variant})  [unwired: 1 in]
        n164 = Enqueue Element(queue=w353, element=w342, error in (no error)=w352) -> (queue out=w340:refnum<queue>, error out=w339:errorcluster)  [unwired: 1 in, 1 out]
      }
      event "Irradiate": Value Change {
        n165 = event-data() -> ("NewVal"=w357:bool)  [unwired: 1 in]
        n166 = To Variant(anything=w362) -> (Variant=w361:variant)
        n167 = Select(t=Consumer_loop_-_States."Irradiation - Check points" ("Consumer loop - States"), s=w357, f=Consumer_loop_-_States."Irradiation - Stop") -> (s? t:f=w355:T4)
        n168 = Bundle("f"=w355, "Variant"=w361) -> (w360:cluster{"f":T4, "Variant":variant})  [unwired: 1 in]
        n169 = Enqueue Element(queue=w364, element=w360, error in (no error)=w363) -> (queue out=w359:refnum<queue>, error out=w358:errorcluster)  [unwired: 1 in, 1 out]
      }
      event "Abort": Value Change {
        n170 = event-data() -> ()  [unwired: 1 in, 1 out]
        n171 = Unbundle By Name(w372) -> ("GPIB Addresses.GPIB Motor"=w371:i16, "GPIB Addresses.GPIB Laser"=w370:string)
        n172 = Flush Queue(queue=w369, error in (no error)=w367) -> (queue out=w368:refnum<queue>, error out=w366:errorcluster)  [unwired: 1 out]
        n173 = call "AB - Abort Motion.vi"("error in"=w374, "Address / Port"=w371) -> ("error out"=w376:errorcluster)  [unwired: 9 in]
        n174 = call "Play laser.vi"("Error In"=w376, "Laser On"=FALSE, "GPIB Address"=w370) -> ("Error Out"=w373:errorcluster)  [unwired: 7 in, 1 out]
      }
      event "Exit": Value Change {
        n175 = event-data() -> ()  [unwired: 1 in, 1 out]
        n176 = Unbundle By Name(w385) -> ("GPIB Addresses.GPIB Motor"=w378:i16, "GPIB Addresses.GPIB Laser"=w383:string)
        n177 = call "ST - Stop motion.vi"("error in"=w380, "Axis"=i8 1, "Address / Port"=w378) -> ("error out"=w379:errorcluster)  [unwired: 6 in, 2 out]
        n178 = call "Play laser.vi"("Error In"=w379, "Laser On"=FALSE, "GPIB Address"=w383) -> ("Error Out"=w384:errorcluster)  [unwired: 7 in, 1 out]
      }
    }
    n179 = Merge Errors(w48, w50) -> (w49:errorcluster)
    n180 = Or(x=w49, y=w52) -> (x .or. y?=w47:bool)
    n181 = call "All close.vi"("Close? (F)"=w47) -> ("Close"=w46:bool)  [unwired: 9 in, 1 out]
  }
  n182 = while "Consumer Loop" {
    tunnel: w17 -> [w392]
    shift-right: [w391] -> _
    shift-left: w16 -> [w390]
    tunnel: w9 -> [w388]
    stop <- w389 stop-if-true
    n183 = case shown="No Error" w390 {
      selector: w390 -> [w396 w778]
      tunnel: w392 -> [w402 _]
      tunnel: [w394 w775] -> w391
      tunnel: [w395 TRUE] -> w389
      tunnel: w388 -> [_ w781]
      frame No Error {
        n184 = Dequeue Element(queue=w402, error in (no error)=w396) -> (queue out=w398:refnum<queue>, element=w401:cluster{"Consumer loop - States":T4, variant}, error out=w399:errorcluster)  [unwired: 1 in, 1 out]
        n185 = Unbundle(w401) -> ("Consumer loop - States"=w400:T4, w397:variant)
        n186 = case shown="\"Move right\"" w400 {
          tunnel: w399 -> [w404 w414 w426 w438 w450 w462 w479 w497 w512 w541 w544 w558 w572 w575 w611 w620 w630 w672 w688 w707 w733 w762 w770]
          tunnel: w398 -> [w405 w415 _ _ _ _ w480 w498 w513 w540 w545 w559 w573 w585 w612 w621 w631 w673 w689 w706 w732 w763 w769]
          tunnel: w397 -> [_ w410 w428 w439 w451 w463 w482 w502 w525 w539 w543 w565 w568 w589 w615 w616 w640 w675 w691 w714 w738 w764 w767]
          tunnel: [w403 w406 w419 w429 w442 w455 w474 w494 w506 w531 w542 w549 w567 w588 w602 w619 w623 w657 w681 w700 w726 w760 w768] -> w394
          frame "Idle", Default {
            n187 = Flush Queue(queue=w405, error in (no error)=w404) -> (error out=w403:errorcluster)  [unwired: 2 out]
          }
          frame "Read Pressure" {
            n188 = Variant To Data(type="" ("Instrument GPIB Addresses.GPIB Laser"), Variant=w410) -> (data=w407:string)  [unwired: 1 in, 1 out]
            n189 = call "Read Pressure.vi"("GPIB Address"=w407) -> ("Pressure [mbar]"=→"Pressure":string)  [unwired: 8 in, 2 out]
            n190 = To Variant(anything=w407) -> (Variant=w412:variant)
            n191 = Bundle("Consumer loop - States"=Consumer_loop_-_States."Read Pressure", "Variant"=w412) -> (w411:T10)  [unwired: 1 in]
            n192 = Wait (ms)(milliseconds to wait=u32 5000) -> ()  [unwired: 1 out]
            n193 = Enqueue Element(queue=w415, element=w411, error in (no error)=w414) -> (error out=w406:errorcluster)  [unwired: 1 in, 2 out]
          }
          frame "Move up" {
            n194 = Variant To Data(error in=w426, type=i16 0 ("Address / Port"), Variant=w428) -> (data=w424:i16, error out=w425:errorcluster)
            n195 = call "VA -Set velocity.vi"("error in"=w425, "Velocity\nset"=20.0 ("Velocity\nset"), "Axis #"=i8 2, "Address / Port"=w424) -> ("error out"=w421:errorcluster, "Address / Port dup"=w420:i16)  [unwired: 4 in, 2 out]
            n196 = call "Step Move.vi"("Error In"=w421, "Delta Y"=300.0 ("Move to travel limit\nset (+ or - )"), "Delta X"=0.0, "Address/Port in"=w420) -> ("Error Out"=w419:errorcluster)  [unwired: 6 in, 1 out]
          }
          frame "Move down" {
            n197 = Variant To Data(error in=w438, type=i16 0 ("Address / Port"), Variant=w439) -> (data=w437:i16, error out=w436:errorcluster)
            n198 = call "VA -Set velocity.vi"("error in"=w436, "Velocity\nset"=20.0 ("Velocity\nset"), "Axis #"=i8 2, "Address / Port"=w437) -> ("error out"=w430:errorcluster, "Address / Port dup"=w431:i16)  [unwired: 4 in, 2 out]
            n199 = call "Step Move.vi"("Error In"=w430, "Delta Y"=-300.0 ("Move to travel limit\nset (+ or - )"), "Delta X"=0.0, "Address/Port in"=w431) -> ("Error Out"=w429:errorcluster)  [unwired: 6 in, 1 out]
          }
          frame "Move left" {
            n200 = Variant To Data(error in=w450, type=i16 0 ("Address / Port"), Variant=w451) -> (data=w448:i16, error out=w449:errorcluster)
            n201 = call "VA -Set velocity.vi"("error in"=w449, "Velocity\nset"=20.0 ("Velocity\nset"), "Axis #"=i8 1, "Address / Port"=w448) -> ("error out"=w441:errorcluster, "Address / Port dup"=w443:i16)  [unwired: 4 in, 2 out]
            n202 = call "Step Move.vi"("Error In"=w441, "Delta Y"=0.0 ("Move to travel limit\nset (+ or - )"), "Delta X"=-300.0, "Address/Port in"=w443) -> ("Error Out"=w442:errorcluster)  [unwired: 6 in, 1 out]
          }
          frame "Move right" {
            n203 = Variant To Data(error in=w462, type=i16 0 ("Address / Port"), Variant=w463) -> (data=w460:i16, error out=w461:errorcluster)
            n204 = call "VA -Set velocity.vi"("error in"=w461, "Velocity\nset"=20.0 ("Velocity\nset"), "Axis #"=i8 1, "Address / Port"=w460) -> ("error out"=w453:errorcluster, "Address / Port dup"=w454:i16)  [unwired: 4 in, 2 out]
            n205 = call "Step Move.vi"("Error In"=w453, "Delta Y"=0.0 ("Move to travel limit\nset (+ or - )"), "Delta X"=300.0, "Address/Port in"=w454) -> ("Error Out"=w455:errorcluster)  [unwired: 6 in, 1 out]
          }
          frame "Move to" {
            w467 = 20.0 ("Velocity\nset")
            n206 = Variant To Data(type=i16 0 ("Instrument GPIB Addresses.GPIB Motor"), Variant=w482) -> (data=w468:i16)  [unwired: 1 in, 1 out]
            n207 = call "VA -Set velocity.vi"("Velocity\nset"=w467, "Axis #"=i8 1, "Address / Port"=w468) -> ("error out"=w469:errorcluster, "Address / Port dup"=w470:i16)  [unwired: 5 in, 2 out]
            n208 = To Variant(anything=w468) -> (Variant=w476:variant)
            n209 = call "VA -Set velocity.vi"("error in"=w469, "Velocity\nset"=w467, "Axis #"=i8 2, "Address / Port"=w470) -> ("error out"=w472:errorcluster, "Address / Port dup"=w471:i16)  [unwired: 4 in, 2 out]
            n210 = Bundle("Consumer loop - States"=Consumer_loop_-_States."Disable buttons", "Variant"=w476) -> (w477:T10)  [unwired: 1 in]
            n211 = Enqueue Element(queue=w480, element=w477, error in (no error)=w479) -> (error out=w475:errorcluster)  [unwired: 1 in, 2 out]
            n212 = call "Go to Move.vi"("Error In"=w472, "Absolute Y"="Absolute Y", "Absolute X"="Absolute X", "Address/Port in"=w471) -> ("Error Out"=w473:errorcluster)  [unwired: 6 in, 1 out]
            n213 = Merge Errors(w475, w473) -> (w474:errorcluster)
          }
          frame "Move Delta" {
            w490 = 20.0 ("Velocity\nset")
            n214 = Variant To Data(type=i16 0 ("Instrument GPIB Addresses.GPIB Motor"), Variant=w502) -> (data=w485:i16)  [unwired: 1 in, 1 out]
            n215 = call "VA -Set velocity.vi"("Velocity\nset"=w490, "Axis #"=i8 1, "Address / Port"=w485) -> ("error out"=w491:errorcluster, "Address / Port dup"=w492:i16)  [unwired: 5 in, 2 out]
            n216 = To Variant(anything=w485) -> (Variant=w496:variant)
            n217 = call "VA -Set velocity.vi"("error in"=w491, "Velocity\nset"=w490, "Axis #"=i8 2, "Address / Port"=w492) -> ("error out"=w487:errorcluster, "Address / Port dup"=w486:i16)  [unwired: 4 in, 2 out]
            n218 = Bundle("Consumer loop - States"=Consumer_loop_-_States."Disable buttons", "Variant"=w496) -> (w499:T10)  [unwired: 1 in]
            n219 = call "Step Move.vi"("Error In"=w487, "Delta Y"="Delta Y", "Delta X"="Delta X", "Address/Port in"=w486) -> ("Error Out"=w493:errorcluster)  [unwired: 6 in, 1 out]
            n220 = Enqueue Element(queue=w498, element=w499, error in (no error)=w497) -> (error out=w495:errorcluster)  [unwired: 1 in, 2 out]
            n221 = Merge Errors(w495, w493) -> (w494:errorcluster)
          }
          frame "Go to calib" {
            w517 = 20.0 ("Velocity\nset")
            n222 = Variant To Data(type=T3 {"GPIB Addresses"={"GPIB Motor"=2, "GPIB Laser"="3"}, "Beam size"={"BeamX"=0.0, "BeamY"=0.0, "Beam Overlap"=0.0}, "Motor speed"={"Xspeed"=0.0, " Yspeed"=0.0}, "Laser parameters"={"Thyratron Bias"=20.0, "Frequency"=0, "Shots/Point"=0.0}, "Irradiation points"={"X1"=0.0, "Y1"=0.0, "X2"=0.0, "Y2"=0.0}, "Calibration Point"={"Xcalib"=0.0, "Ycalib"=0.0}} ("User Interface data"), Variant=w525) -> (data=w516:T3)  [unwired: 1 in, 1 out]
            n223 = Unbundle By Name(w516) -> ("GPIB Addresses.GPIB Motor"=w510:i16)
            n224 = Unbundle By Name(w516) -> ("Calibration Point.Xcalib"=w515:dbl, "Calibration Point.Ycalib"=w514:dbl)
            n225 = call "VA -Set velocity.vi"("Velocity\nset"=w517, "Axis #"=i8 1, "Address / Port"=w510) -> ("error out"=w520:errorcluster, "Address / Port dup"=w521:i16)  [unwired: 5 in, 2 out]
            n226 = To Variant(anything=w510) -> (Variant=w509:variant)
            n227 = call "VA -Set velocity.vi"("error in"=w520, "Velocity\nset"=w517, "Axis #"=i8 2, "Address / Port"=w521) -> ("error out"=w523:errorcluster, "Address / Port dup"=w522:i16)  [unwired: 4 in, 2 out]
            n228 = Bundle("Consumer loop - States"=Consumer_loop_-_States."Disable buttons", "Variant"=w509) -> (w508:T10)  [unwired: 1 in]
            n229 = call "Go to Move.vi"("Error In"=w523, "Absolute Y"=w514, "Absolute X"=w515, "Address/Port in"=w522) -> ("Error Out"=w505:errorcluster)  [unwired: 6 in, 1 out]
            n230 = Enqueue Element(queue=w513, element=w508, error in (no error)=w512) -> (error out=w507:errorcluster)  [unwired: 1 in, 2 out]
            n231 = Merge Errors(w507, w505) -> (w506:errorcluster)
          }
          frame "Stop Motion" {
            n232 = Variant To Data(type=i16 0 ("GPIB Addresses.GPIB Motor"), Variant=w539) -> (data=w537:i16)  [unwired: 1 in, 1 out]
            n233 = call "ST - Stop motion.vi"("Axis"=i8 1, "Address / Port"=w537) -> ("error out"=w530:errorcluster, "Address / Port dup"=w529:i16)  [unwired: 7 in, 1 out]
            n234 = call "ST - Stop motion.vi"("error in"=w530, "Axis"=i8 2, "Address / Port"=w529) -> ("error out"=w528:errorcluster)  [unwired: 6 in, 2 out]
            n235 = To Variant(anything=-1) -> (Variant=w535:variant)
            n236 = Bundle("Consumer loop - States"=Consumer_loop_-_States."Idle", "Variant"=w535) -> (w533:T10)  [unwired: 1 in]
            n237 = Enqueue Element(queue=w540, element=w533, error in (no error)=w541) -> (error out=w532:errorcluster)  [unwired: 1 in, 2 out]
            n238 = Merge Errors(w532, w528) -> (w531:errorcluster)
          }
          frame "Disable buttons" {
            w548 = T7."Disabled and Grayed Out" ("Disabled")
            n239 = property on="Move" class="Bool"("DisabledEnum"=w548) -> ()  [unwired: 2 in, 2 out]
            n240 = property on="Right" class="Bool (strict)"("DisabledEnum"=w548) -> ()  [unwired: 2 in, 2 out]
            n241 = property on="Left" class="Bool (strict)"("DisabledEnum"=w548) -> ()  [unwired: 2 in, 2 out]
            n242 = property on="Up" class="Bool (strict)"("DisabledEnum"=w548) -> ()  [unwired: 2 in, 2 out]
            n243 = property on="Down" class="Bool (strict)"("DisabledEnum"=w548) -> ()  [unwired: 2 in, 2 out]
            n244 = Bundle("Consumer loop - States"=Consumer_loop_-_States."Check if move done", w543) -> (w546:cluster{"Consumer loop - States":T4, variant})  [unwired: 1 in]
            n245 = Enqueue Element(queue=w545, element=w546, error in (no error)=w544) -> (error out=w542:errorcluster)  [unwired: 1 in, 2 out]
          }
          frame "Check if move done" {
            n246 = Variant To Data(type=i16 0 ("Address / Port"), Variant=w565) -> (data=w551:i16)  [unwired: 1 in, 1 out]
            n247 = call "MD - Read motion done status.vi"("Axis"=i8 1, "Address / Port"=w551) -> ("Done"=w561:bool, "Address / Port dup"=w562:i16)  [unwired: 6 in, 2 out]
            n248 = call "MD - Read motion done status.vi"("Axis"=i8 2, "Address / Port"=w562) -> ("Done"=w560:bool)  [unwired: 6 in, 3 out]
            n249 = To Variant(anything=w551) -> (Variant=w550:variant)
            n250 = And(x=w560, y=w561) -> (x .and. y?=w557:bool)
            n251 = Select(t=Consumer_loop_-_States."Enable buttons" ("Consumer loop - States"), s=w557, f=Consumer_loop_-_States."Check if move done") -> (s? t:f=w554:T4)
            n252 = Bundle("f"=w554, "Variant"=w550) -> (w555:cluster{"f":T4, "Variant":variant})  [unwired: 1 in]
            n253 = Wait (ms)(milliseconds to wait=u32 100) -> ()  [unwired: 1 out]
            n254 = Enqueue Element(queue=w559, element=w555, error in (no error)=w558) -> (error out=w549:errorcluster)  [unwired: 1 in, 2 out]
          }
          frame "Enable buttons" {
            w569 = T7."Enabled" ("Disabled")
            n255 = property on="Move" class="Bool"("DisabledEnum"=w569) -> ()  [unwired: 2 in, 2 out]
            n256 = property on="Right" class="Bool (strict)"("DisabledEnum"=w569) -> ()  [unwired: 2 in, 2 out]
            n257 = property on="Left" class="Bool (strict)"("DisabledEnum"=w569) -> ()  [unwired: 2 in, 2 out]
            n258 = property on="Up" class="Bool (strict)"("DisabledEnum"=w569) -> ()  [unwired: 2 in, 2 out]
            n259 = property on="Down" class="Bool (strict)"("DisabledEnum"=w569) -> ()  [unwired: 2 in, 2 out]
            n260 = Bundle("Consumer loop - States"=Consumer_loop_-_States."Idle", w568) -> (w571:cluster{"Consumer loop - States":T4, variant})  [unwired: 1 in]
            n261 = Enqueue Element(queue=w573, element=w571, error in (no error)=w572) -> (error out=w567:errorcluster)  [unwired: 1 in, 2 out]
          }
          frame "Irradiation - Stop" {
            n262 = Variant To Data(type=T3 {"GPIB Addresses"={"GPIB Motor"=2, "GPIB Laser"="3"}, "Beam size"={"BeamX"=0.0, "BeamY"=0.0, "Beam Overlap"=0.0}, "Motor speed"={"Xspeed"=0.0, " Yspeed"=0.0}, "Laser parameters"={"Thyratron Bias"=20.0, "Frequency"=1, "Shots/Point"=1.0}, "Irradiation points"={"X1"=0.0, "Y1"=0.0, "X2"=0.0, "Y2"=0.0}, "Calibration Point"={"Xcalib"=0.0, "Ycalib"=0.0}} ("User Interface data"), Variant=w589) -> (data=w579:T3)  [unwired: 1 in, 1 out]
            n263 = Unbundle By Name(w579) -> ("GPIB Addresses.GPIB Motor"=w577:i16, "GPIB Addresses.GPIB Laser"=w578:string)
            n264 = Flush Queue(queue=w585, error in (no error)=w575) -> (queue out=w576:refnum<queue>, error out=w574:errorcluster)  [unwired: 1 out]
            n265 = call "Play laser.vi"("Laser On"=FALSE, "GPIB Address"=w578) -> ("Error Out"=w580:errorcluster)  [unwired: 8 in, 1 out]
            n266 = call "ST - Stop motion.vi"("error in"=w580, "Axis"=i8 1, "Address / Port"=w577) -> ("error out"=w595:errorcluster, "Address / Port dup"=w594:i16)  [unwired: 6 in, 1 out]
            n267 = To Variant(anything=-1) -> (Variant=w582:variant)
            n268 = call "ST - Stop motion.vi"("error in"=w595, "Axis"=i8 2, "Address / Port"=w594) -> ("error out"=w586:errorcluster)  [unwired: 6 in, 2 out]
            n269 = Bundle("Consumer loop - States"=Consumer_loop_-_States."Irradiation - Enable buttons", "Variant"=w582) -> (w584:T10)  [unwired: 1 in]
            n270 = Enqueue Element At Opposite End(queue=w576, element=w584, error in (no error)=w574) -> (error out=w587:errorcluster)  [unwired: 1 in, 2 out]
            n271 = Merge Errors(w587, w586) -> (w588:errorcluster)
          }
          frame "Irradiation - Check points" {
            n272 = Variant To Data(type=T3 {"GPIB Addresses"={"GPIB Motor"=2, "GPIB Laser"="3"}, "Beam size"={"BeamX"=0.0, "BeamY"=0.0, "Beam Overlap"=0.0}, "Motor speed"={"Xspeed"=0.0, " Yspeed"=0.0}, "Laser parameters"={"Thyratron Bias"=20.0, "Frequency"=1, "Shots/Point"=1.0}, "Irradiation points"={"X1"=0.0, "Y1"=0.0, "X2"=0.0, "Y2"=0.0}, "Calibration Point"={"Xcalib"=0.0, "Ycalib"=0.0}} ("User Interface data"), Variant=w615) -> (data=w609:T3)  [unwired: 1 in, 1 out]
            n273 = Unbundle By Name(w609) -> ("Irradiation points.X2"=w608:dbl, "Irradiation points.X1"=w607:dbl, "Irradiation points.Y2"=w605:dbl, "Irradiation points.Y1"=w606:dbl)
            n274 = Greater Or Equal?(x=w608, y=w607) -> (x >= y?=w604:bool)
            n275 = Less Or Equal?(x=w605, y=w606) -> (x <= y?=w603:bool)
            n276 = And(x=w604, y=w603) -> (x .and. y?=w597:bool)
            n277 = To Variant(anything=w609) -> (Variant=w610:variant)
            n278 = Not(x=w597) -> (.not. x?=w596:bool)
            n279 = Select(t=Consumer_loop_-_States."Irradiation - Disable buttons" ("Consumer loop - States"), s=w597, f=Consumer_loop_-_States."Idle") -> (s? t:f=w599:T4)
            n280 = Bundle("f"=w599, "Variant"=w610) -> (w613:cluster{"f":T4, "Variant":variant})  [unwired: 1 in]
            n281 = call "Display Message to User"("Enable"=w596, "Message"="Error!\nCheck the position of your points") -> ()  [unwired: 8 in, 2 out]
            n282 = Enqueue Element(queue=w612, element=w613, error in (no error)=w611) -> (error out=w602:errorcluster)  [unwired: 1 in, 2 out]
          }
          frame "Irradiation - Disable buttons" {
            w622 = T7."Disabled and Grayed Out" ("Disabled")
            n283 = property on="Move" class="Bool"("DisabledEnum"=w622) -> ()  [unwired: 2 in, 2 out]
            n284 = property on="Right" class="Bool (strict)"("DisabledEnum"=w622) -> ()  [unwired: 2 in, 2 out]
            n285 = property on="Left" class="Bool (strict)"("DisabledEnum"=w622) -> ()  [unwired: 2 in, 2 out]
            n286 = property on="Up" class="Bool (strict)"("DisabledEnum"=w622) -> ()  [unwired: 2 in, 2 out]
            n287 = property on="Down" class="Bool (strict)"("DisabledEnum"=w622) -> ()  [unwired: 2 in, 2 out]
            n288 = Bundle("Consumer loop - States"=Consumer_loop_-_States."Irradiation - Init position", w616) -> (w618:cluster{"Consumer loop - States":T4, variant})  [unwired: 1 in]
            n289 = Enqueue Element(queue=w621, element=w618, error in (no error)=w620) -> (error out=w619:errorcluster)  [unwired: 1 in, 2 out]
          }
          frame "Irradiation - Init position" {
            n290 = Variant To Data(type=T3 {"GPIB Addresses"={"GPIB Motor"=2, "GPIB Laser"="3"}, "Beam size"={"BeamX"=0.0, "BeamY"=0.0, "Beam Overlap"=0.0}, "Motor speed"={"Xspeed"=0.0, " Yspeed"=0.0}, "Laser parameters"={"Thyratron Bias"=20.0, "Frequency"=1, "Shots/Point"=1.0}, "Irradiation points"={"X1"=0.0, "Y1"=0.0, "X2"=0.0, "Y2"=0.0}, "Calibration Point"={"Xcalib"=0.0, "Ycalib"=0.0}} ("User Interface data"), Variant=w640) -> (data=w626:T3)  [unwired: 1 in, 1 out]
            n291 = Unbundle By Name(w626) -> ("GPIB Addresses.GPIB Laser"=w637:string, "GPIB Addresses.GPIB Motor"=w638:i16)
            n292 = Unbundle By Name(w626) -> ("Irradiation points.X1"=w636:dbl, "Irradiation points.Y1"=w635:dbl, "Laser parameters.Thyratron Bias"=w633:dbl, "Laser parameters.Frequency"=w634:u16)
            n293 = call "VA -Set velocity.vi"("Velocity\nset"=20.0 ("Velocity\nset"), "Axis #"=i8 1, "Address / Port"=w638) -> ("error out"=w645:errorcluster, "Address / Port dup"=w644:i16)  [unwired: 5 in, 2 out]
            n294 = Bundle("Thyratron Bias"=w633, "Frequency"=w634) -> (w632:cluster{"Thyratron Bias":dbl, "Frequency":u16})  [unwired: 1 in]
            n295 = To Variant(anything=w626) -> (Variant=w627:variant)
            n296 = call "VA -Set velocity.vi"("error in"=w645, "Velocity\nset"=20.0 ("Velocity\nset"), "Axis #"=i8 2, "Address / Port"=w644) -> ("error out"=w643:errorcluster, "Address / Port dup"=w642:i16)  [unwired: 4 in, 2 out]
            n297 = call "PA -Move to absolute position.vi"("Move to absolute\nposition - set"=w636, "error in"=w643, "Axis #"=i8 1, "Address / Port"=w642) -> ("error out"=w651:errorcluster, "Address / Port dup"=w650:i16)  [unwired: 2 in, 2 out]
            n298 = call "PA -Move to absolute position.vi"("Move to absolute\nposition - set"=w635, "error in"=w651, "Axis #"=i8 2, "Address / Port"=w650) -> ("error out"=w641:errorcluster)  [unwired: 2 in, 3 out]
            n299 = Bundle("Consumer loop - States"=Consumer_loop_-_States."Irradiation - Check if done", "Variant"=w627) -> (w629:T10)  [unwired: 1 in]
            n300 = call "Laser setup.vi"("Error In"=w641, "Laser Parameters"=w632, "GPIB Address"=w637) -> ("Error Out"=w625:errorcluster)  [unwired: 7 in, 1 out]
            n301 = Enqueue Element(queue=w631, element=w629, error in (no error)=w630) -> (error out=w624:errorcluster)  [unwired: 1 in, 2 out]
            n302 = Merge Errors(w624, w625) -> (w623:errorcluster)
          }
          frame "Irradiation - Check if done" {
            n303 = Variant To Data(type=T3 {"GPIB Addresses"={"GPIB Motor"=2, "GPIB Laser"="3"}, "Beam size"={"BeamX"=0.0, "BeamY"=0.0, "Beam Overlap"=0.0}, "Motor speed"={"Xspeed"=0.0, " Yspeed"=0.0}, "Laser parameters"={"Thyratron Bias"=20.0, "Frequency"=1, "Shots/Point"=1.0}, "Irradiation points"={"X1"=0.0, "Y1"=0.0, "X2"=0.0, "Y2"=0.0}, "Calibration Point"={"Xcalib"=0.0, "Ycalib"=0.0}} ("User Interface data"), Variant=w675) -> (data=w660:T3)  [unwired: 1 in, 1 out]
            n304 = Unbundle By Name(w660) -> ("GPIB Addresses.GPIB Motor"=w667:i16)
            n305 = call "MD - Read motion done status.vi"("Axis"=i8 1, "Address / Port"=w667) -> ("error out"=w668:errorcluster, "Done"=w663:bool, "Address / Port dup"=w671:i16)  [unwired: 6 in, 1 out]
            n306 = call "MD - Read motion done status.vi"("error in"=w668, "Axis"=i8 2, "Address / Port"=w671) -> ("error out"=w655:errorcluster, "Done"=w662:bool)  [unwired: 5 in, 2 out]
            n307 = To Variant(anything=w660) -> (Variant=w659:variant)
            n308 = And(x=w662, y=w663) -> (x .and. y?=w666:bool)
            n309 = Select(t=Consumer_loop_-_States."Irradiation - Sweep X", s=w666, f=Consumer_loop_-_States."Irradiation - Check if done" ("Consumer loop - States")) -> (s? t:f=w661:T4)
            n310 = Bundle("Consumer loop - States"=w661, "Variant"=w659) -> (w658:T10)  [unwired: 1 in]
            n311 = Wait (ms)(milliseconds to wait=u32 100) -> ()  [unwired: 1 out]
            n312 = Enqueue Element(queue=w673, element=w658, error in (no error)=w672) -> (error out=w656:errorcluster)  [unwired: 1 in, 2 out]
            n313 = Merge Errors(w656, w655) -> (w657:errorcluster)
          }
          frame "Irradiation - Sweep X" {
            n314 = Variant To Data(type=T3 {"GPIB Addresses"={"GPIB Motor"=2, "GPIB Laser"="3"}, "Beam size"={"BeamX"=0.0, "BeamY"=0.0, "Beam Overlap"=0.0}, "Motor speed"={"Xspeed"=0.0, " Yspeed"=0.0}, "Laser parameters"={"Thyratron Bias"=20.0, "Frequency"=1, "Shots/Point"=1.0}, "Irradiation points"={"X1"=0.0, "Y1"=0.0, "X2"=0.0, "Y2"=0.0}, "Calibration Point"={"Xcalib"=0.0, "Ycalib"=0.0}} ("User Interface data"), Variant=w691) -> (data=w679:T3)  [unwired: 1 in, 1 out]
            n315 = Unbundle By Name(w679) -> ("GPIB Addresses.GPIB Motor"=w685:i16, "GPIB Addresses.GPIB Laser"=w686:string)
            n316 = Unbundle By Name(w679) -> ("Motor speed.Xspeed"=w678:dbl, "Irradiation points.X2"=w677:dbl, "Irradiation points.X1"=w676:dbl)
            n317 = call "Play laser.vi"("Laser On"=TRUE, "GPIB Address"=w686) -> ("Error Out"=w698:errorcluster)  [unwired: 8 in, 1 out]
            n318 = To Variant(anything=w679) -> (Variant=w687:variant)
            n319 = call "VA -Set velocity.vi"("error in"=w698, "Velocity\nset"=w678, "Axis #"=i8 1, "Address / Port"=w685) -> ("error out"=w694:errorcluster, "Axis # dup"=w695:i8, "Address / Port dup"=w696:i16)  [unwired: 4 in, 1 out]
            n320 = Subtract(x=w677, y=w676) -> (x-y=w697:dbl)
            n321 = call "PR - Move to relative position.vi"("error in"=w694, "Nstep"=w697, "Axis  #"=w695, "Address / Port"=w696) -> ("error out"=w680:errorcluster)  [unwired: 3 in, 2 out]
            n322 = Bundle("Consumer loop - States"=Consumer_loop_-_States."Irradiation - Check X", "Variant"=w687) -> (w683:T10)  [unwired: 1 in]
            n323 = Enqueue Element(queue=w689, element=w683, error in (no error)=w688) -> (error out=w682:errorcluster)  [unwired: 1 in, 2 out]
            n324 = Merge Errors(w682, w680) -> (w681:errorcluster)
          }
          frame "Irradiation - Check X" {
            n325 = Variant To Data(type=T3 {"GPIB Addresses"={"GPIB Motor"=2, "GPIB Laser"="3"}, "Beam size"={"BeamX"=0.0, "BeamY"=0.0, "Beam Overlap"=0.0}, "Motor speed"={"Xspeed"=0.0, " Yspeed"=0.0}, "Laser parameters"={"Thyratron Bias"=20.0, "Frequency"=1, "Shots/Point"=1.0}, "Irradiation points"={"X1"=0.0, "Y1"=0.0, "X2"=0.0, "Y2"=0.0}, "Calibration Point"={"Xcalib"=0.0, "Ycalib"=0.0}} ("User Interface data"), Variant=w714) -> (data=w705:T3)  [unwired: 1 in, 1 out]
            n326 = Unbundle By Name(w705) -> ("GPIB Addresses.GPIB Motor"=w713:i16)
            n327 = call "MD - Read motion done status.vi"("Axis"=i8 1, "Address / Port"=w713) -> ("error out"=w699:errorcluster, "Done"=w709:bool)  [unwired: 6 in, 2 out]
            n328 = To Variant(anything=w705) -> (Variant=w704:variant)
            n329 = Select(t=Consumer_loop_-_States."Irradiation - Check Y" ("Consumer loop - States"), s=w709, f=Consumer_loop_-_States."Irradiation - Check X") -> (s? t:f=w702:T4)
            n330 = Bundle("f"=w702, "Variant"=w704) -> (w703:cluster{"f":T4, "Variant":variant})  [unwired: 1 in]
            n331 = Enqueue Element(queue=w706, element=w703, error in (no error)=w707) -> (error out=w701:errorcluster)  [unwired: 1 in, 2 out]
            n332 = Wait (ms)(milliseconds to wait=u32 100) -> ()  [unwired: 1 out]
            n333 = Merge Errors(w701, w699) -> (w700:errorcluster)
          }
          frame "Irradiation - Check Y" {
            # "#debugged? Testare un po'"
            n334 = Variant To Data(type=T3 {"GPIB Addresses"={"GPIB Motor"=2, "GPIB Laser"="3"}, "Beam size"={"BeamX"=0.0, "BeamY"=0.0, "Beam Overlap"=0.0}, "Motor speed"={"Xspeed"=0.0, " Yspeed"=0.0}, "Laser parameters"={"Thyratron Bias"=20.0, "Frequency"=1, "Shots/Point"=1.0}, "Irradiation points"={"X1"=0.0, "Y1"=0.0, "X2"=0.0, "Y2"=0.0}, "Calibration Point"={"Xcalib"=0.0, "Ycalib"=0.0}} ("User Interface data"), Variant=w738) -> (data=w731:T3)  [unwired: 1 in, 1 out]
            n335 = Unbundle By Name(w731) -> ("GPIB Addresses.GPIB Motor"=w719:i16, "GPIB Addresses.GPIB Laser"=w737:string)
            n336 = Unbundle By Name(w731) -> ("Beam size.BeamY"=w723:dbl, "Beam size.Beam Overlap"=w724:dbl, "Irradiation points.Y2"=w725:dbl)
            n337 = call "Play laser.vi"("Laser On"=FALSE, "GPIB Address"=w737) -> ("Error Out"=w720:errorcluster)  [unwired: 8 in, 1 out]
            n338 = call "TP - Read actual position.vi"("error in"=w720, "Axis"=i8 2, "Address / Port"=w719) -> ("error out"=w716:errorcluster, "Query the current actual\nposition - read"=w717:dbl)  [unwired: 5 in, 2 out]
            n339 = Subtract(x=w723, y=w724) -> (x-y=w722:dbl)
            n340 = To Variant(anything=w731) -> (Variant=w730:variant)
            n341 = Subtract(x=w717, y=w722) -> (x-y=w721:dbl)
            n342 = Greater Or Equal?(x=w721, y=w725) -> (x >= y?=w736:bool)
            n343 = Select(t=Consumer_loop_-_States."Irradiation - Sweep Y" ("Consumer loop - States"), s=w736, f=Consumer_loop_-_States."Irradiation - Enable buttons") -> (s? t:f=w728:T4)
            n344 = Bundle("f"=w728, "Variant"=w730) -> (w729:cluster{"f":T4, "Variant":variant})  [unwired: 1 in]
            n345 = Enqueue Element(queue=w732, element=w729, error in (no error)=w733) -> (error out=w727:errorcluster)  [unwired: 1 in, 2 out]
            n346 = Merge Errors(w727, w716) -> (w726:errorcluster)
          }
          frame "Irradiation - Sweep Y" {
            n347 = Variant To Data(type=T3 {"GPIB Addresses"={"GPIB Motor"=2, "GPIB Laser"="3"}, "Beam size"={"BeamX"=0.0, "BeamY"=0.0, "Beam Overlap"=0.0}, "Motor speed"={"Xspeed"=0.0, " Yspeed"=0.0}, "Laser parameters"={"Thyratron Bias"=20.0, "Frequency"=1, "Shots/Point"=1.0}, "Irradiation points"={"X1"=0.0, "Y1"=0.0, "X2"=0.0, "Y2"=0.0}, "Calibration Point"={"Xcalib"=0.0, "Ycalib"=0.0}} ("User Interface data"), Variant=w764) -> (data=w755:T3)  [unwired: 1 in, 1 out]
            n348 = Unbundle By Name(w755) -> ("Beam size.BeamY"=w753:dbl, "Beam size.Beam Overlap"=w754:dbl, "Irradiation points.X1"=w745:dbl)
            n349 = Unbundle By Name(w755) -> ("GPIB Addresses.GPIB Motor"=w756:i16)
            n350 = Subtract(x=w753, y=w754) -> (x-y=w742:dbl)
            n351 = Negate(x=w742) -> (-x=w741:dbl)
            n352 = To Variant(anything=w755) -> (Variant=w758:variant)
            n353 = call "PR - Move to relative position.vi"("Nstep"=w741, "Axis  #"=i8 2, "Address / Port"=w756) -> ("error out"=w750:errorcluster, "Address / Port dup"=w749:i16)  [unwired: 4 in, 1 out]
            n354 = call "VA -Set velocity.vi"("error in"=w750, "Velocity\nset"=20.0 ("Velocity\nset"), "Axis #"=i8 1, "Address / Port"=w749) -> ("error out"=w746:errorcluster, "Address / Port dup"=w747:i16)  [unwired: 4 in, 2 out]
            n355 = Bundle("Consumer loop - States"=Consumer_loop_-_States."Irradiation - Check if done", "Variant"=w758) -> (w759:T10)  [unwired: 1 in]
            n356 = call "PA -Move to absolute position.vi"("Move to absolute\nposition - set"=w745, "error in"=w746, "Axis #"=i8 1, "Address / Port"=w747) -> ("error out"=w744:errorcluster)  [unwired: 2 in, 3 out]
            n357 = Enqueue Element(queue=w763, element=w759, error in (no error)=w762) -> (error out=w761:errorcluster)  [unwired: 1 in, 2 out]
            n358 = Merge Errors(w761, w744) -> (w760:errorcluster)
          }
          frame "Irradiation - Enable buttons" {
            w774 = T7."Enabled" ("Disabled")
            n359 = property on="Move" class="Bool"("DisabledEnum"=w774) -> ()  [unwired: 2 in, 2 out]
            n360 = property on="Right" class="Bool (strict)"("DisabledEnum"=w774) -> ()  [unwired: 2 in, 2 out]
            n361 = property on="Left" class="Bool (strict)"("DisabledEnum"=w774) -> ()  [unwired: 2 in, 2 out]
            n362 = To Variant(anything=w767) -> (Variant=w771:variant)
            n363 = property on="Up" class="Bool (strict)"("DisabledEnum"=w774) -> ()  [unwired: 2 in, 2 out]
            n364 = property on="Down" class="Bool (strict)"("DisabledEnum"=w774) -> ()  [unwired: 2 in, 2 out]
            n365 = local write "Irradiate"(FALSE ("Irradiate")) -> ()
            n366 = Bundle("Consumer loop - States"=Consumer_loop_-_States."Idle", "Variant"=w771) -> (w773:T10)  [unwired: 1 in]
            n367 = Enqueue Element(queue=w769, element=w773, error in (no error)=w770) -> (error out=w768:errorcluster)  [unwired: 1 in, 2 out]
          }
        }
        n368 = Unbundle By Name(w394) -> ("status"=w393:bool)
        n369 = call "All close.vi"("Close? (F)"=w393) -> ("Close"=w395:bool)  [unwired: 9 in, 1 out]
      }
      frame Error {
        n370 = Unbundle By Name(w781) -> ("GPIB Addresses.GPIB Motor"=w777:i16, "GPIB Addresses.GPIB Laser"=w776:string)
        n371 = call "AB - Abort Motion.vi"("error in"=w778, "Address / Port"=w777) -> ("error out"=w780:errorcluster)  [unwired: 9 in]
        n372 = call "Play laser.vi"("Error In"=w780, "Laser On"=FALSE, "GPIB Address"=w776) -> ("Error Out"=w775:errorcluster)  [unwired: 7 in, 1 out]
      }
    }
  }
  n373 = call <vilib>:"IMAQdx Close Camera.vi"("error in"=w24, "Session In"=w25) -> ()  [unwired: 9 in, 1 out]
  n374 = Release Queue(queue=w11, error in (no error)=w12) -> ()  [unwired: 1 in, 3 out]
